vi "Compute Optimal IRF v3.vi"(8 "Error In":errorcluster, 9 "IRF Optimization Control":T1={"Search Range"=1e-18, "Search Step"=1e-18, "Tail Threshold (%)"=1e-09, "Regularized IRF"=FALSE, "Export Plot"=FALSE, "Export Data"=FALSE, "Smooth Metrics"=FALSE, "S-G Side Points"=1, "S-G Polynomial Order"=3, "Metrics"=enum."Average"} {"S-G Polynomial Order" min=3 max=10; "S-G Side Points" min=1; "Tail Threshold (%)" min=0.0 max=100.0; "Search Range" min=0.0 max=1e-09}, 11 "Selected Plot Info":T3={"Multiplot XY Graph"=refnum, "Mouse Coordinates"={"Horizontal"=0, "Vertical"=0}, "Plot Index"=-1}) -> (0 "Error Out":errorcluster, 1 "Optimal Tau":dbl, 2 "Plot Name":string, 3 "IRF Plot":cluster{"X Array":dbl[], "Y Array":dbl[]}, 4 "Optimal IRF Results String":string, 5 "Optimization Graph":cluster{dbl[], dbl[]}[](graph))   [LabVIEW 2021, in "Fits.lvlib"]
doc: "Extract IRF from provided decay and time constant"
uses:
  Fits.lvlib
  Graphs/XY Graph/XY Graph Selected Plot Info.ctl
  Graphs/XY Graph/XY Graph Refnum.ctl
  <vilib>/Utility/miscctls.llb/LVPoint32TypeDef.ctl
  AlliGator/AlliGator IRF Optimization Controls.ctl
  AlliGator/AlliGator IRF Deconvolution Metrics.ctl
  AlliGator/AlliGator Settings List.ctl
  IRF(X)PSED Extraction Options.ctl
  Fourier Series Smoothing Option.ctl
  Fourier Series Truncation.ctl
  IRF Extraction Method.ctl
  Fit Plot Request Information.ctl
  <vilib>/Utility/miscctls.llb/LVPointDoubleTypeDef.ctl
  Fit Models.ctl
  cc3fc4cb-3fe6-4f43-9f61-aa3a5ef9d036.vi
  <vilib>/Analysis/1siggen.llb/Ramp Pattern by Delta.vi
  <userlib>/_OpenG.lib/array/array.llb/Filter 1D Array with Scalar (DBL)__ogtk.vi
  <userlib>/_OpenG.lib/array/array.llb/Delete Elements from 1D Array (DBL)__ogtk.vi
  <vilib>/Analysis/NI_AALBase.lvlib
  AlliGator/AlliGator Settings.lvlib
  Time/Time.lvlib
  Utilities/Utilities.lvlib
  Arrays/Arrays.lvlib
  Graphs/XY Graph/XY Graph Add-Ons.lvlib
  <vilib>/Analysis/NI_AALPro.lvlib
  <userlib>/_OpenG.lib/array/array.llb/openg_array.lvlib
  AlliGator/AlliGator IRF.lvlib
panel:
  in  "Display":bool
  out "# Tail Points":i32
  out "min value":dbl
  in  "Debug":bool
  out "IRF Graph":cluster{"X Array":dbl[], "Y Array":dbl[]}[](graph)
  out "Current Tau (ns)":dbl format="%#_4g"
  # "1. In debug mode, move the cursor in the Optimiztion Graph to display the corresponding IRF in the IRF Graph\n2. Click on the close window X to stop debugging"
  # "see the AlliGator License on the block diagram (Ctrl+E or Window:Show Block Diagram)"
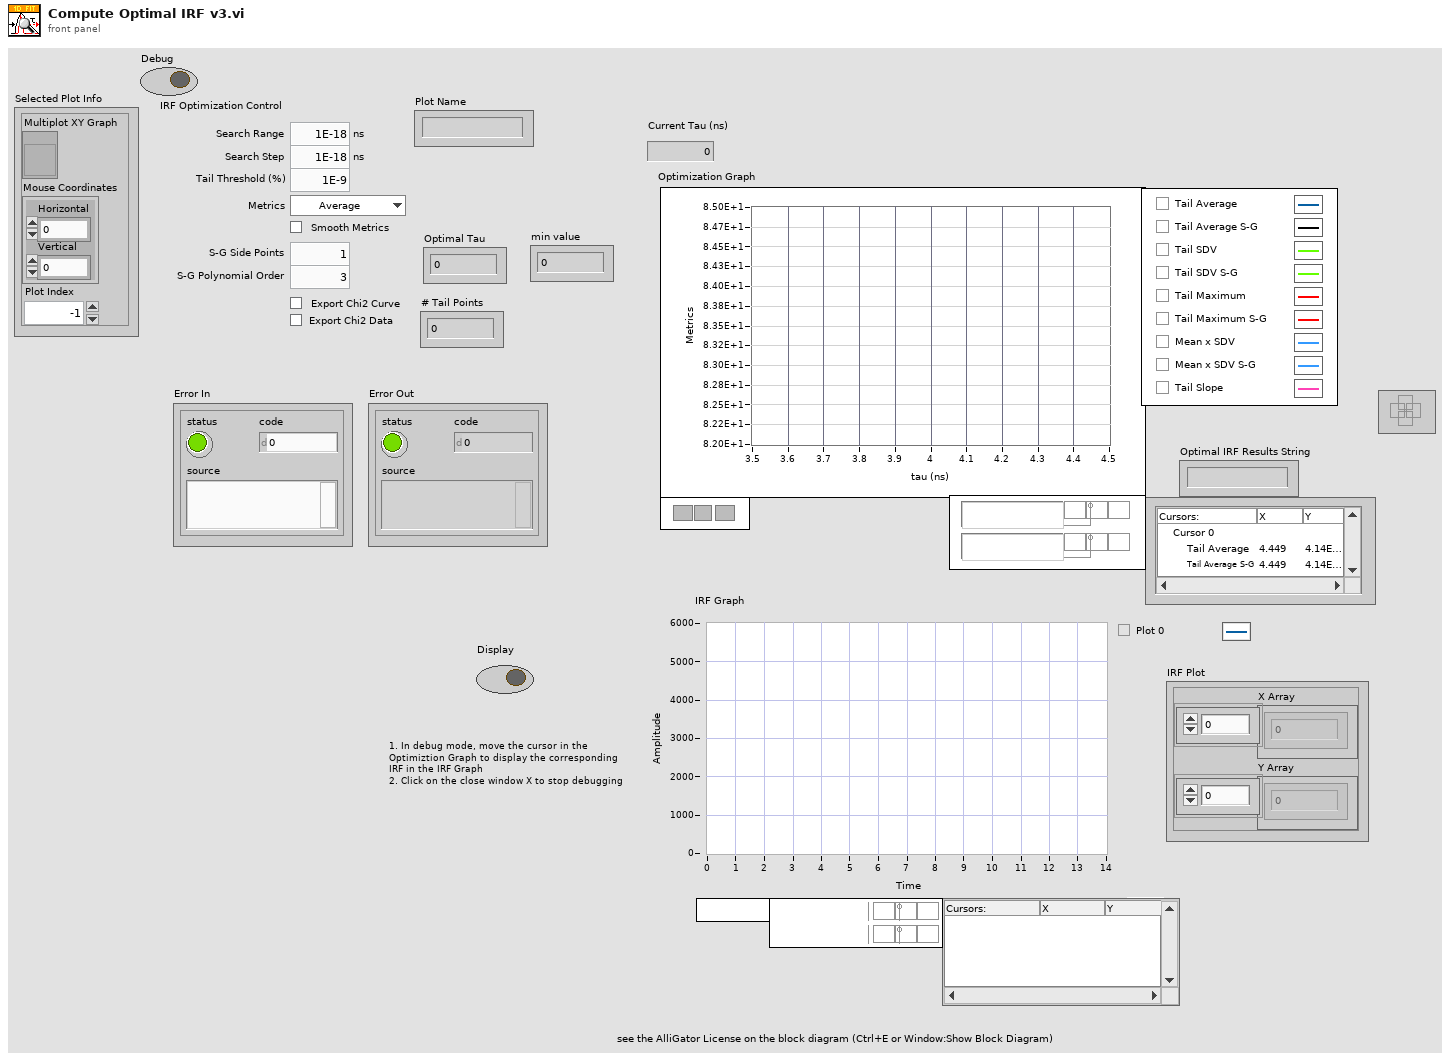
[diagram p1: front panel]
types:
  T1 = typedef "AlliGator Decay Analysis.lvlib/AlliGator IRF.lvlib/AlliGator IRF Optimization Controls.ctl" = cluster{"Search Range":dbl[unit], "Search Step":dbl[unit], "Tail Threshold (%)":dbl, "Regularized IRF":bool, "Export Plot":bool, "Export Data":bool, "Smooth Metrics":bool, "S-G Side Points":i32, "S-G Polynomial Order":i32, "Metrics":T2}
  T2 = typedef "AlliGator Decay Analysis.lvlib/AlliGator IRF.lvlib/AlliGator IRF Deconvolution Metrics.ctl" = enum16{"Average", "SDV", "Max", "Average * SDV", "Slope"}
  T3 = typedef "XY Graph Add-Ons.lvlib/XY Graph Selected Plot Info.ctl" = cluster{"Multiplot XY Graph":T4, "Mouse Coordinates":T5, "Plot Index":i32}
  T4 = typedef "XY Graph Add-Ons.lvlib/XY Graph Refnum.ctl" = refnum<vi>
  T5 = typedef "LVPoint32TypeDef.ctl" = cluster{"Horizontal":i32, "Vertical":i32}
  T6 = typedef "Fits.lvlib/IRF Extraction Method.ctl" = enum16{"Direct", "Topless", "Toeplitz"}
  T7 = typedef "AlliGator Settings.lvlib/AlliGator Settings List.ctl" = enum16{"GUI:Visible Settings Tab", "GUI:Last Run Version", "Source Image:Use Image Histogram for Contrast", "Source Image:Low Count Pixels Rejection Options", "Source Image:High Count Pixels Rejection Options", "Source Image:Use Image Brightness", "Source Image:Blend Overlay with Image Background", "Source Image:Use Fixed ROI Diameter", "Source Image:ROI Diameter", "Source Image:ROI Center Color", "Source Image:Peak Threshold", "Source Image:Intensity Threshold", "Source Image:Image Binning Options", "Source Image:Image Smoothing Options", "Source Image:Image Histogram Active", "Source Image:Invert Binary Mask", "Source Image:Hot Pixel Removal", "Source Image:Overlay Analyzed ROI Center", "Source Image:Auto-Adjust Contrast", "Source Image:Histogram Lower Percentile", "Source Image:Histogram Upper Percentile", "Source Image:Save Source Image", "Source Image:Scale Bar Options", "Source Image:Image Resolution (Pixel Size)", "Source Image:Flatfield Correction", "Source Image:Show Dead Left Columns Correction", "Source Image:Dead Left Columns Correction", "Source Image:Image Pre-Processing Operations Order", "Data Information:Gate Width", "Data Information:Nanotime Gate Separation", "Data Information:Macrotime Gate Separation", "Data Information:Gate Step", "Data Information:# Gates", "Data Information:Gate Image Exposure", "Data Information:Gate Image Integration", "Data Information:Gates to Skip", "Data Information:Gates to Keep", "Data Information:Define Gates to", "Data Information:Channel Name", "Data Information:Available Channel Names", "Data Information:Channel Arithmetic", "Data Information:Background File Subtraction", "Data Information:Background File", "Data Information:Background Scaling Factor", "Data Information:Background Pile-up Correction", "Data Information:Background Pixel Well Capacity", "Data Information:Laser Period", "Data Information:SYNC Period", "Data Information:Pile-up Correction", "Data Information:Pixel Well Capacity", "Data Information:Dataset Scaling Factor", "Fluorescence Decay_Decay Pre-Processing:Reverse Gates", "Fluorescence Decay_Decay Pre-Processing:Verbose Decay Pre-Processing", "Fluorescence Decay_Decay Pre-Processing:Use Decay Pre-Processing", "Fluorescence Decay_Decay Pre-Processing:Background Subtraction", "Fluorescence Decay_Decay Pre-Processing:Background Definition Range", "Fluorescence Decay_Decay Pre-Processing:Baseline Subtraction Method", "Fluorescence Decay_Decay Pre-Processing:Decay Pre-Processing Operations Order", "Fluorescence Decay_Decay Pre-Processing:Smoothing Parameter", "Fluorescence Decay_Decay Pre-Processing:Shift Decay", "Fluorescence Decay_Decay Pre-Processing:Decay Shift Parameters", "Fluorescence Decay_Decay Pre-Processing:Fold Decay", "Fluorescence Decay_Decay Pre-Processing:# Folds", "Fluorescence Decay_Decay Pre-Processing:1-Normalize Decay", "Fluorescence Decay_Decay Pre-Processing:[0-1]-Normalize Decay", "Fluorescence Decay_Decay Pre-Processing:Smoothen Decay", "Fluorescence Decay_Decay Pre-Processing:Extrapolate Decay", "Fluorescence Decay_Decay Pre-Processing:Use Periodicity", "Fluorescence Decay_Decay Pre-Processing:Use Cursors", "Fluorescence Decay_Decay Pre-Processing:Tail Fraction", "Fluorescence Decay_Decay Pre-Processing:Head Fraction", "Fluorescence Decay_Decay Pre-Processing:Additional Points", "Fluorescence Decay_Decay Pre-Processing:Straighten Decay", "Fluorescence Decay_Decay Pre-Processing:Constant Background", "Fluorescence Decay_Decay Pre-Processing:Pixel-Normalize Decay", "Fluorescence Decay_Advanced Analysis:Extract IRF instead of Decay", "Fluorescence Decay_Advanced Analysis:IRF Extraction Options", "Fluorescence Decay_Advanced Analysis:IRF Optimization Options", "Fluorescence Decay_Advanced Analysis:Square Pulse Options", "Fluorescence Decay_Advanced Analysis:IRF Order", "Fluorescence Decay_Advanced Analysis:IRF Time Constants", "Fluorescence Decay_Advanced Analysis:Wavelet Analysis Options", "Fluorescence Decay_Advanced Analysis:Average Lifetime Options", "Fluorescence Decay_Fit Options:Fit Options", "Fluorescence Decay_Fit Options:Use Legacy Fitting Approach", "Fluorescence Decay_Fit Options:Use Data Information Laser Period", "Fluorescence Decay_Fit Parameters:Displayed Fit Parameters", "Fluorescence Decay_Fit Parameters:Fit Parameter Constraints", "Fluorescence Decay_Fit Parameters:Export Tabulated Results", "Fluorescence Decay_Fit Parameters:MLE Baseline Offset Type", "Fluorescence Decay_Fit Parameters:MLE Baseline Offset", "Fluorescence Decay_Fit Parameters:Guess Parameter Names", "Fluorescence Decay_Fit Parameters:Guess Parameter Values", "Fluorescence Decay_Fit Parameters:Guess Parameters Options", "Fluorescence Decay_Styles:Show Last Decay Only", "Fluorescence Decay_Styles:Decay Graph Color Array", "Fluorescence Decay:Decay Graph Active", "Fluorescence Decay Statistics:Min Peak Value", "Fluorescence Decay Statistics:Reject Low Decay Peak Pixels", "Fluorescence Decay Statistics:Reject High Decay Peak Pixels", "Fluorescence Decay Statistics:Max Peak Value", "Time Traces:Use File Timestamp", "Time Traces:Time Step", "Time Traces:Use Intensity Correction File", "Time Traces:Intensity Correction File", "Phasor Plot:Phasor Plot Smoothing Options", "Phasor Plot:Phasor Plot Size", "Phasor Plot:Phasor Plot Graphics Options", "Phasor Plot:Cumulative Phasor Plot", "Phasor Plot:Use Phasor Brightness", "Phasor Plot:Blend Overlay with Phasor Background", "Phasor Plot:Save Phasor Plot", "Phasor Plot:Show References", "Phasor Plot:Phasor Ratio Decay Range", "Phasor Plot:Exponential Fading", "Phasor Plot:Phasor Ratio Reference Colors", "Phasor Plot:Reference Radius", "Phasor Plot:Show Color Map Vertices", "Phasor Plot:Phasor Plot Active", "Phasor Plot:Phasor Ratio Color Map Type", "Phasor Plot:Phasor Ratio Color Map", "Phasor Plot:Phasor Ratio Display Range", "Phasor Plot:Selected Image ROI(s)", "Phasor Plot:All Image ROIs", "Phasor Plot:Selected Phasor Plot ROI(s)", "Phasor Plot:All Phasor Plot ROIs", "Phasor Plot:Phasor Ratio Color-Coded Quantity", "Phasor Plot:Store Phasor Harmonics", "Phasor Plot:Draw Reference Segment", "Phasor Plot:User-Defined Quantity", "Phasor Graph:Phasor Frequency", "Phasor Graph:Phasor Ratio Type", "Phasor Graph:Pixel-level Phasor Computation", "Phasor Graph:Save Phasor Graph", "Phasor Graph:Phasor Graph Active", "Phasor Graph:Phasor SDV Options", "Phasor Calibration:Use Backup Calibration if needed", "Phasor Graph:Define Shortest Lifetime as", "Phasor Calibration:Backup Calibration Type", "Phasor Calibration:Calibration Type", "Phasor Calibration:Calibration Lifetime", "Phasor Calibration:Calibration Map Algorithm", "Single-Exponential Phasor Locus (SEPL):Gate Parameters", "Single-Exponential Phasor Locus (SEPL):User-defined Gate", "Single-Exponential Phasor Locus (SEPL):User-defined IRF", "Single-Exponential Phasor Locus (SEPL):Phasor Parameters", "Single-Exponential Phasor Locus (SEPL):Decay & IRF Parameters", "Single-Exponential Phasor Locus (SEPL):Display Parameters", "Lifetime Analysis:Decay Analysis Parameters", "Lifetime Analysis:Lifetime Map Active", "Plugins:Python Settings", "Miscellaneous:Verbose Mode", "Miscellaneous:Beep after Script", "Miscellaneous:Saved Image File Format", "Miscellaneous:Exported Gate Image Settings", "Miscellaneous:Include Loading in Timing", "Miscellaneous:Verbose Settings Mode", "Miscellaneous:Histogram Options", "Miscellaneous:Beep on Error", "Miscellaneous:# Logical Processors Used", "Miscellaneous:ROI Description Max Characters", "Miscellaneous:Verbose Error Mode", "Miscellaneous:Transparent Mask Color"}
  T8 = typedef "Fits.lvlib/IRF(X)PSED Extraction Options.ctl" = cluster{"Time Constant for IRF Extraction":dbl[unit], "IRF Order":i32, "Fourier Series Smoothing":T9, "Noise Threshold":dbl, "Smoothing Width":dbl, "Fourier Series Truncation":T10, "Truncation Order":i32, "Save Power Spectrum":bool, "Smoothing":bool, "Smoothing Parameter":dbl, "Smoothing Order":u32, "Method":T6}
  T9 = typedef "Fits.lvlib/Fourier Series Smoothing Option.ctl" = enum16{"None", "Lanczos Factors", "Fejer Summation"}
  T10 = typedef "Fits.lvlib/Fourier Series Truncation.ctl" = enum16{"Automatic", "Fixed"}
  T11 = typedef "Fits.lvlib/Fit Plot Request Information.ctl" = cluster{"XY Graph Ref":refnum<vi>, "Mouse Coordinates":T12, "Fit Model":T13, "Plot Index":i32}
  T12 = typedef "LVPointDoubleTypeDef.ctl" = cluster{"X":dbl, "Y":dbl}
  T13 = typedef "Fits.lvlib/Fit Models.ctl" = enum16{"Select a Fit Model...", "           Single Peak", "Gaussian", "Asymmetric Gaussian", "Lorentzian", "Asymmetric Lorentzian", "Gaussian/Lorentzian", "Lorentzian/Gaussian", "           Double Peak", "Two Gaussians", "Two Asymmetric Gaussians", "Two H-Connected Gaussians", "Two T-Connected Gaussians", "Two H-Connected Asymmetric Gaussians", "Two T-Connected Asymmetric Gaussians", "           Triple Peak", "Three Gaussians", "Three Asymmetric Gaussians", "              Decays", "1-Exponential", "IRF*PSED", "2-Exponentials", "               ACF", "2D Gaussian ACF", "2D Gaussian + Blinking ACF", "2D Gaussian + Flow ACF", "3D Gaussian ACF", "3D Gaussian + Blinking ACF", "             Multiplot", "2D Gaussian ACF & 2D Gaussian + Flow ACF"}
  T14 = typedef "XY Graph Add-Ons.lvlib/XY Plot Data.ctl" = cluster{"X Array":dbl[], "Y Array":dbl[]}
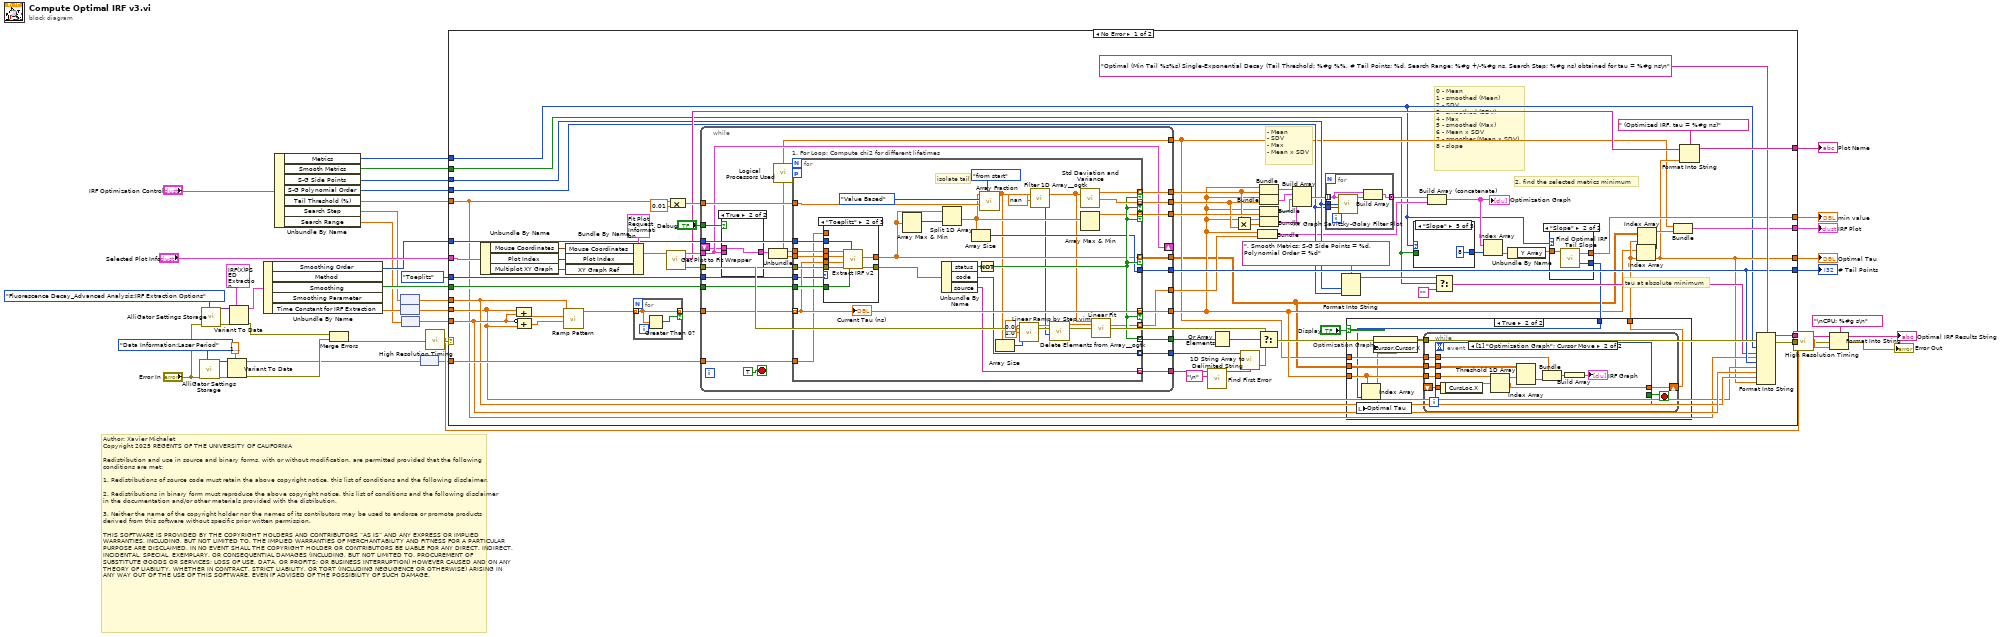
[diagram p0: block diagram]
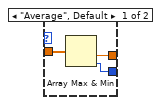
[diagram p2: hidden frame]
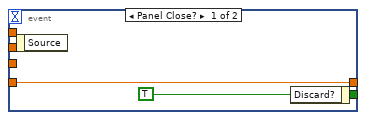
[diagram p4: hidden frame]
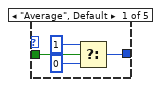
[diagram p5: hidden frame]
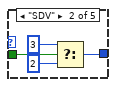
[diagram p6: hidden frame]
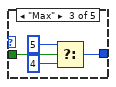
[diagram p7: hidden frame]
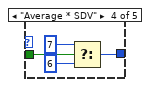
[diagram p8: hidden frame]
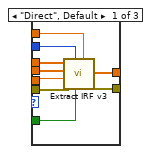
[diagram p9: hidden frame]
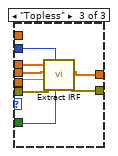
[diagram p10: hidden frame]
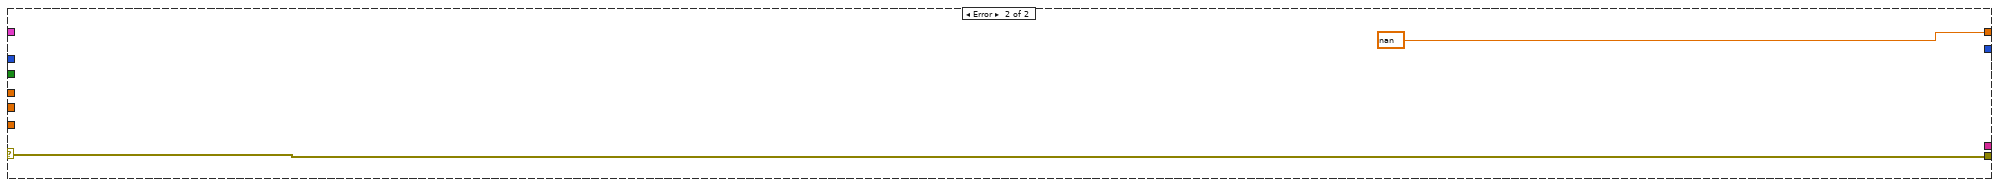
[diagram p12: hidden frame]
diagram:
  # "Author: Xavier Michalet\nCopyright 2025 REGENTS OF THE UNIVERSITY OF CALIFORNIA\n\nRedistribution and use in source and binary forms, with or without modification, are permitted provided that the following conditions are met:\n\n1. Redistributions of source code must retain the above copyright notice, this list of conditions and the following disclaimer.\n\n2. Redistributions in binary form must reproduce the above copyright notice, this list of conditions and the following disclaimer in the documentation and/or other materials provided with the distribution.\n\n3. Neither the name of the copyright holder nor the names of its contributors may be used to endorse or promote products derived from this software without specific prior written permission.\n\nTHIS SOFTWARE IS PROVIDED BY THE COPYRIGHT HOLDERS AND CONTRIBUTORS “AS IS” AND ANY EXPRESS OR IMPLIED WARRANTIES, INCLUDING, BUT NOT LIMITED TO, THE IMPLIED WARRANTIES OF MERCHANTABILITY AND FITNESS FOR A PARTICULAR PURPOSE ARE DISCLAIMED. IN NO EVENT SHALL THE COPYRIGHT HOLDER OR CONTRIBUTORS BE LIABLE FOR ANY DIRECT, INDIRECT, INCIDENTAL, SPECIAL, EXEMPLARY, OR CONSEQUENTIAL DAMAGES (INCLUDING, BUT NOT LIMITED TO, PROCUREMENT OF SUBSTITUTE GOODS OR SERVICES; LOSS OF USE, DATA, OR PROFITS; OR BUSINESS INTERRUPTION) HOWEVER CAUSED AND ON ANY THEORY OF LIABILITY, WHETHER IN CONTRACT, STRICT LIABILITY, OR TORT (INCLUDING NEGLIGENCE OR OTHERWISE) ARISING IN ANY WAY OUT OF THE USE OF THIS SOFTWARE, EVEN IF ADVISED OF THE POSSIBILITY OF SUCH DAMAGE."
  n1 = call "AlliGator Settings Storage.vi"("AlliGator Settings List"=AlliGator_Settings_List."Data Information:Laser Period", "Error In"="Error In") -> ("Error Out"=w18:errorcluster, "Variant Data out"=w20:variant)  [unwired: 8 in]
  n2 = call "AlliGator Settings Storage.vi"("AlliGator Settings List"=AlliGator_Settings_List."Fluorescence Decay_Advanced Analysis:IRF Extraction Options", "Error In"="Error In") -> ("Error Out"=w37:errorcluster, "Variant Data out"=w43:variant)  [unwired: 8 in]
  n3 = Variant To Data(error in=w18, type=dbl[unit] 1e-09 ("Time Constant"), Variant=w20) -> (data=w15:dbl[unit], error out=w16:errorcluster)
  n4 = Variant To Data(error in=w37, type=T8 {"Time Constant for IRF Extraction"=1e-18, "IRF Order"=1, "Fourier Series Smoothing"=enum."None", "Noise Threshold"=0.0, "Smoothing Width"=0.0, "Fourier Series Truncation"=enum."Automatic", "Truncation Order"=0, "Save Power Spectrum"=FALSE, "Smoothing"=FALSE, "Smoothing Parameter"=0.0, "Smoothing Order"=1, "Method"=enum."Direct"} ("IRF Extraction Options"), Variant=w43) -> (data=w44:T8, error out=w36:errorcluster)
  n5 = Unbundle By Name(w44) -> ("Smoothing Order"=w25:u32, "Smoothing"=w24:bool, "Time Constant for IRF Extraction"=w27:dbl[unit])  [unwired: 2 out]
  n6 = Unbundle By Name("IRF Optimization Control") -> ("Metrics"=w1:T2, "Smooth Metrics"=w4:bool, "S-G Side Points"=w3:i32, "S-G Polynomial Order"=w2:i32, "Tail Threshold (%)"=w12:dbl, "Search Step"=w11:dbl[unit], "Search Range"=w8:dbl[unit])
  n7 = Merge Errors(w36, w16) -> (w17:errorcluster)
  n8 = node(w11) -> (w40:dbl)
  n9 = node(w27) -> (w39:dbl)
  n10 = node(w8) -> (w7:dbl)
  n11 = node(w15) -> (w14:dbl)
  n12 = call "High Resolution Timing.vi"("Error In"=w17) -> ("elapsed (relative) seconds"=w35:dbl, "Error Out"=w41:errorcluster)  [unwired: 16 in, 1 out]
  n13 = case shown="No Error" w41 {
    selector: w41 -> [_ w257]
    tunnel: [w100 w257] -> w45
    tunnel: w39 -> [w73 _]
    tunnel: w40 -> [w79 _]
    tunnel: w7 -> [w80 _]
    tunnel: "Selected Plot Info" -> [w115 _]
    tunnel: [w101 _] -> w34
    tunnel: [w58 _] -> w26
    tunnel: w25 -> [w108 _]
    tunnel: w24 -> [w107 _]
    tunnel: [w54 nan] -> w23
    tunnel: [w103 _] -> w22
    tunnel: w12 -> [w67 _]
    tunnel: IRF_Extraction_Method."Toeplitz" ("Method") -> [w99 _]
    tunnel: w14 -> [w98 _]
    tunnel: [w76 _] -> w6
    tunnel: [w74 _] -> w5
    tunnel: w4 -> [w48 _]
    tunnel: w3 -> [w64 _]
    tunnel: w2 -> [w63 _]
    tunnel: w1 -> [w46 _]
    frame No Error {
      # "0 - Mean\n1 - smoothed (Mean)\n2 - SDV\n3 - smoothed (SDV)\n4 - Max\n5 - smoothed (Max)\n6 - Mean x SDV\n7 - smoother (Mean x SDV)\n8 - slope"
      # "- Mean\n- SDV\n- Max\n- Mean x SDV"
      # "tau at absolute minimum"
      # "2. find the selected metrics minimum"
      n14 = Unbundle By Name(w115) -> ("Mouse Coordinates"=w112:T5, "Plot Index"=w111:i32, "Multiplot XY Graph"=w113:T4)
      n15 = Compound Arithmetic op=ADD(w73, w80) -> (w117:dbl)
      n16 = Compound Arithmetic op=ADD(invert w80, w73) -> (w116:dbl)
      n17 = call-poly <vilib>:"Ramp Pattern.vi"("start"=w116, "end"=w117, "delta"=w79) -> ("Ramp Pattern"=w78:dbl[])  [unwired: 6 in, 2 out]
      n18 = Bundle By Name(cluster=T11 {"XY Graph Ref"=refnum, "Mouse Coordinates"={"X"=0.0, "Y"=0.0}, "Fit Model"=enum."IRF*PSED", "Plot Index"=-1} ("Fit Plot Information"), "Mouse Coordinates"=w112, "Plot Index"=w111, "XY Graph Ref"=w113) -> (w109:T11)
      n19 = for {
        tunnel: w78 -> [w166] mode=indexing
        tunnel: [w166] -> w77 mode=indexing if=w165
        n20 = Greater Than 0?(x=w166) -> (x > 0?=w165:bool)
      }
      n21 = call "Get Plot to Fit Wrapper.vi"("Fit Plot Information"=w109) -> ("error out"=w94:errorcluster, "Plot Name"=w72:string, "Plot"=w110:T14)  [unwired: 5 in, 3 out]
      n22 = Compound Arithmetic op=MULTIPLY(w67, 0.01 ("value")) -> (w87:dbl)
      n23 = while {
        tunnel: w110 -> [w172]
        tunnel: [w190] -> w47
        tunnel: w108 -> [w189]
        tunnel: w107 -> [w188]
        tunnel: w77 -> [w187]
        tunnel: w99 -> [w186]
        tunnel: w98 -> [w185]
        tunnel: [w184] -> w97
        tunnel: w94 -> [w183]
        tunnel: [w182] -> w93
        tunnel: [w181] -> w92
        tunnel: w87 -> [w180]
        tunnel: [w179] -> w85
        tunnel: [w178] -> w51
        tunnel: [w177] -> w83
        tunnel: [w176] -> w75
        tunnel: "Debug" -> [w174]
        shift-right: [w172] -> _
        shift-left: _ -> [w170]
        tunnel: [w169] -> w74
        tunnel: [w168] -> w50
        tunnel: [w167] -> w55
        stop <- TRUE stop-if-true
        n24 = case shown="True" w174 {
          tunnel: w172 -> [w249 _]
          tunnel: [w249 w250] -> w171
          tunnel: w170 -> [_ w250]
          frame False {
          }
          frame True {
          }
        }
        n25 = Unbundle(w171) -> ("X Array"=w168:dbl[], "Y Array"=w173:dbl[])
        n26 = call "Logical Processors Used.vi"() -> ("# Logical Processor Used"=w191:i32)  [unwired: 6 in]
        n27 = for "1. For Loop: Compute chi2 for different lifetimes" {
          tunnel: w187 -> [w217] mode=indexing
          workers-P: w191 -> [_]
          tunnel: w168 -> [w221]
          tunnel: w173 -> [w223]
          tunnel: w183 -> [w222]
          tunnel: [w201] -> w190 mode=indexing if=w208
          tunnel: w189 -> [w220]
          tunnel: w188 -> [w219]
          tunnel: [w218] -> w176 mode=indexing if=w208
          tunnel: [w217] -> w178 mode=indexing if=w208
          tunnel: w180 -> [w207]
          tunnel: w186 -> [w215]
          tunnel: w185 -> [w214]
          tunnel: [w208] -> w184 mode=indexing
          tunnel: [w212] -> w182 mode=indexing
          tunnel: [w211] -> w181 mode=indexing
          tunnel: [w210] -> w177 mode=indexing if=w208
          tunnel: [w202] -> w179 mode=indexing if=w208
          tunnel: [w206] -> w169
          tunnel: [w200] -> w167 mode=indexing
          # "isolate tail"
          n28 = case shown="\"Toeplitz\"" w215 {
            tunnel: w223 -> [w231 w240 w247]
            tunnel: w222 -> [w229 w239 w246]
            tunnel: w221 -> [w232 w238 w248]
            tunnel: w220 -> [w226 w237 w241]
            tunnel: w219 -> [w225 w236 w242]
            tunnel: [w227 w235 w244] -> w201
            tunnel: [w228 w234 w243] -> w213
            tunnel: w217 -> [w230 w233 w245]
            tunnel: w214 -> [w224 _ _]
            frame "Direct", Default {
              n29 = call "Extract IRF v3.vi"("Period"=w224, "Tail Smoothing (T)"=w225, "Smoothing Order"=w226, "Error In"=w229, "Time Constant"=w230, "Intensity Array"=w231, "t Array"=w232) -> ("Error Out"=w228:errorcluster, "IRF Array"=w227:dbl[])  [unwired: 1 in, 2 out]
            }
            frame "Toeplitz" {
              n30 = call "Extract IRF v2.vi"("Tail Smoothing (T)"=w236, "Smoothing Order"=w237, "Error In"=w239, "Time Constant"=w233, "Intensity Array"=w240, "t Array"=w238) -> ("Error Out"=w234:errorcluster, "IRF Array"=w235:dbl[])  [unwired: 2 in, 2 out]
            }
            frame "Topless" {
              n31 = call "Extract IRF.vi"("Tail Smoothing (T)"=w242, "Smoothing Order"=w241, "Error In"=w246, "Time Constant"=w245, "Intensity Array"=w247, "t Array"=w248) -> ("Error Out"=w243:errorcluster, "IRF Array"=w244:dbl[])  [unwired: 2 in, 2 out]
            }
          }
          n32 = Array Max & Min(array=w201) -> (max index (indices)=w209:i32)  [unwired: 3 out]
          n33 = Unbundle By Name(w213) -> ("status"=w216:bool, "code"=w212:i32, "source"=w211:string)
          n34 = Split 1D Array(array=w201, index=w209) -> (second subarray=w203:dbl[])  [unwired: 1 out]
          n35 = Array Size(array=w203) -> (size(s)=w206:i32)
          n36 = Not(x=w216) -> (.not. x?=w208:bool)
          n37 = call "Array Fraction.vi"("Direction (from start)"=enum16{"from start", "from end"}."from start", "fraction [0, 1]"=w207, "Method (Length Based)"=enum16{"Value Based", "Length Based"}."Value Based", "Array"=w203) -> ("Array out"=w196:dbl[])  [unwired: 6 in, 1 out]
          n38 = Array Size(array=w196) -> (size(s)=w195:i32)
          n39 = call "Linear Ramp by Step.vim"("# Elements (1)"=w195, "Step (1)"=1.0, "Start (0)"=0.0) -> ("Ramp"=w194:dbl[])  [unwired: 8 in]
          n40 = call-poly <userlib>:"Filter 1D Array__ogtk.vi"("items to filter"=nan, "array"=w196) -> ("filtered item indices"=w192:i32[])  [unwired: 4 in, 1 out]
          n41 = call-poly <userlib>:"Delete Elements from Array__ogtk.vi"("indices"=w192, "array"=w194) -> ("array w/ subset deleted"=w193:dbl[])  [unwired: 8 in, 1 out]
          n42 = call <vilib>:"Std Deviation and Variance.vi"("X"=w196) -> ("mean"=w210:dbl, "standard deviation"=w218:dbl)  [unwired: 1 in, 1 out]
          n43 = Array Max & Min(array=w203) -> (max value=w202:dbl)  [unwired: 3 out]
          n44 = call <vilib>:"Linear Fit.vi"("Y"=w196, "X"=w193) -> ("slope"=w200:dbl)  [unwired: 9 in, 4 out]
          "Current Tau (ns)" <- w217
        }
      }
      n45 = call <vilib>:"1D String Array to Delimited String.vi"("delimiter"="\n", "string array"=w92) -> ("delimited string"=w91:string)  [unwired: 9 in]
      n46 = Or Array Elements(Boolean array=w97) -> (logical OR=w96:bool)
      n47 = Multiply(x=w83, y=w75) -> (x*y=w82:dbl[])
      n48 = call <vilib>:"Find First Error.vi"("source messages"=w91, "error codes"=w93) -> ("error out"=w89:errorcluster)  [unwired: 2 in, 1 out]
      n49 = Bundle(w51, w55) -> (w49:cluster{dbl[], dbl[]})  [unwired: 1 in]
      n50 = Bundle(w51, w83) -> (w106:cluster{dbl[], dbl[]})  [unwired: 1 in]
      n51 = Bundle(w51, w75) -> (w105:cluster{dbl[], dbl[]})  [unwired: 1 in]
      n52 = Bundle(w51, w85) -> (w88:cluster{dbl[], dbl[]})  [unwired: 1 in]
      n53 = Bundle(w51, w82) -> (w84:cluster{dbl[], dbl[]})  [unwired: 1 in]
      n54 = Select(t=w94, s=w96, f=w89) -> (s? t:f=w95:errorcluster)
      n55 = Build Array(w106, w105, w88, w84) -> (w71:cluster{dbl[], dbl[]}[])
      n56 = for {
        tunnel: w71 -> [w253] mode=indexing
        tunnel: [w254] -> w70 mode=concatenating
        tunnel: w64 -> [w252]
        tunnel: w63 -> [w251]
        n57 = call "XY Graph Savitzky-Golay Filter Plot.vi"("polynomial order  (3)"=w251, "side points (6)"=w252, "Plot in"=w253) -> ("Plot out"=w255:cluster{"X Array":dbl[], "Y Array":dbl[]})  [unwired: 7 in, 1 out]
        n58 = Build Array(w253, w255) -> (w254:cluster{"X Array":dbl[], "Y Array":dbl[]}[])
      }
      n59 = Format Into String(format string=", Smooth Metrics: S-G Side Points = %d, Polynomial Order = %d" ("initial string"), w64, w63) -> (resulting string=w65:string)  [unwired: 2 in, 1 out]
      n60 = case shown="\"Slope\"" w46 {
        tunnel: w48 -> [w151 w155 w159 w163 _]
        tunnel: [w148 w152 w156 w160 8 ("f")] -> w60
        frame "Average", Default {
          n61 = Select(t=1, s=w151, f=0) -> (s? t:f=w148:i32)
        }
        frame "SDV" {
          n62 = Select(t=3, s=w155, f=2) -> (s? t:f=w152:i32)
        }
        frame "Max" {
          n63 = Select(t=5, s=w159, f=4) -> (s? t:f=w156:i32)
        }
        frame "Average * SDV" {
          n64 = Select(t=7, s=w163, f=6) -> (s? t:f=w160:i32)
        }
        frame "Slope" {
        }
      }
      n65 = Build Array (concatenate)(w70, w49) -> (w56:cluster{"X Array":dbl[], "Y Array":dbl[]}[])
      "Optimization Graph" <- w56
      n66 = Select(t=w65, s=w48, f="") -> (s? t:f=w61:string)
      n67 = Index Array(array=w56, index=w60) -> (element=w69:cluster{"X Array":dbl[], "Y Array":dbl[]})
      n68 = Unbundle By Name(w69) -> ("Y Array"=w68:dbl[])
      n69 = case shown="\"Slope\"" w46 {
        tunnel: [w120 w122] -> w76
        tunnel: w68 -> [w119 w123]
        tunnel: [w118 w121] -> w53
        frame "Average", Default {
          n70 = Array Max & Min(array=w119) -> (min value=w120:dbl, min index (indices)=w118:i32)  [unwired: 2 out]
        }
        frame "Slope" {
          n71 = call "Find Optimal IRF Tail Slope.vi"("Slope Array"=w123) -> ("Optimal Index"=w121:i32, "Optimal Slope"=w122:dbl)  [unwired: 9 in]
        }
      }
      n72 = case shown="True" "Display" {
        tunnel: w51 -> [_ w127]
        tunnel: w47 -> [_ w131]
        tunnel: w53 -> [w124 w126]
        tunnel: [w124 w129] -> w52
        tunnel: w50 -> [_ w130]
        frame False {
        }
        frame True {
          n73 = Index Array(array=w127, index=w126) -> (element=w125:dbl)
          n74 = local write "Optimal Tau"(w125) -> ()
          n75 = property on="Optimization Graph" class="XYGraph (strict)"("Cursor.Cursor X"=w125) -> (error out=w128:errorcluster)  [unwired: 2 in, 1 out]
          n76 = while {
            tunnel: w127 -> [w136]
            tunnel: w131 -> [w135]
            tunnel: w130 -> [w134]
            shift-right: [w133] -> w129
            shift-left: _ -> [w132]
            tunnel: w128 -> [_]
            stop <- w137 stop-if-true
            n77 = event shown="[1] \"Optimization Graph\": Cursor Move" {
              selector: _ -> [_ _]
              dyn-events: _ -> [_ _]
              timeout: _ -> [_ _]
              tunnel: [w139 _] -> w137
              tunnel: w136 -> [_ w144]
              tunnel: w135 -> [_ w146]
              tunnel: w134 -> [_ w141]
              tunnel: [w138 w140] -> w133
              tunnel: w132 -> [w138 _]
              event Panel Close? {
                w139 = TRUE ("Discard?")
                n78 = event-data() -> ()  [unwired: 1 in, 1 out]
                n79 = event-data("Discard?"=w139) -> ()  [unwired: 1 in, 1 out]
              }
              event "Optimization Graph": Cursor Move {
                n80 = event-data() -> ("CursLoc.X"=w147:dbl)  [unwired: 1 in]
                n81 = Threshold 1D Array(2:w147, 3:w144) -> (0:w140:dbl)  [unwired: 1 in]
                n82 = Index Array(array=w146, index (row)=w140) -> (element=w145:dbl[])  [unwired: 1 in]
                n83 = Bundle("X Array"=w141, "IRF Array"=w145) -> (w143:cluster{"X Array":dbl[], "IRF Array":dbl[]})  [unwired: 1 in]
                n84 = Build Array(w143) -> (→"IRF Graph":cluster{"X Array":dbl[], "IRF Array":dbl[]}[])
              }
            }
          }
        }
      }
      n85 = Index Array(array=w51, index=w52) -> (element=w54:dbl)
      n86 = Index Array(array=w47, index (row)=w52) -> (element=w59:dbl[])  [unwired: 1 in]
      n87 = Bundle("X Array"=w50, "IRF Array"=w59) -> (w58:cluster{"X Array":dbl[], "IRF Array":dbl[]})  [unwired: 1 in]
      n88 = Format Into String(format string=" (Optimized IRF, tau = %#g ns)", initial string=w72, w54) -> (resulting string=w103:string)  [unwired: 1 in, 1 out]
      n89 = Format Into String(format string="Optimal (Min Tail %s%s) Single-Exponential Decay (Tail Threshold: %#g %%, # Tail Points: %d, Search Range: %#g +/-%#g ns, Search Step: %#g ns) obtained for tau = %#g ns\n" ("string"), error in=w95, w46, w61, w67, w74, w73, w80, w79, w54) -> (resulting string=w101:string, error out=w100:errorcluster)  [unwired: 1 in]
    }
    frame Error {
    }
  }
  "Optimal Tau" <- w23
  "Plot Name" <- w22
  "IRF Plot" <- w26
  "min value" <- w6
  "# Tail Points" <- w5
  n90 = call "High Resolution Timing.vi"("relative seconds (NaN)"=w35, "Error In"=w45) -> ("elapsed (relative) seconds"=w32:dbl, "Error Out"=w30:errorcluster)  [unwired: 15 in, 1 out]
  n91 = Format Into String(format string="\nCPU: %#g s\n", initial string=w34, error in=w30, w32) -> (resulting string=→"Optimal IRF Results String":string, error out=→"Error Out":errorcluster)
